vi "002 Case calculadora strings.vi"() -> ()   [LabVIEW 2019]
panel:
  out "Resultat":dbl
  in  "Selector d'operació":u8(slide) scale=0.0..3.0
  in  "Nombre 1":dbl
  in  "Nombre 2":dbl
  # "CALCULADORA"
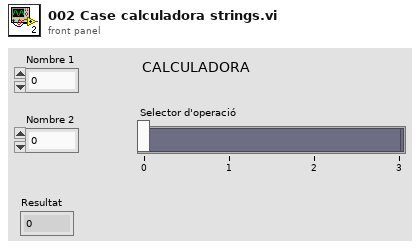
[diagram p1: front panel]
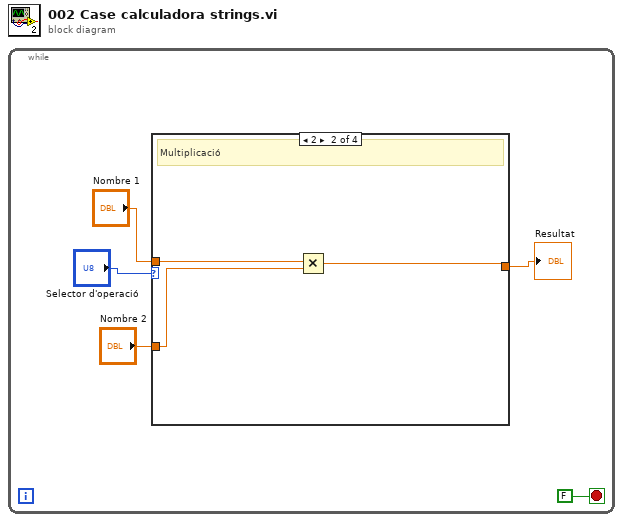
[diagram p0: block diagram]
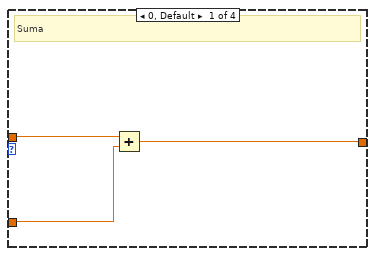
[diagram p2: hidden frame]
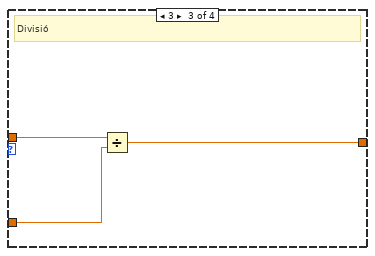
[diagram p3: hidden frame]
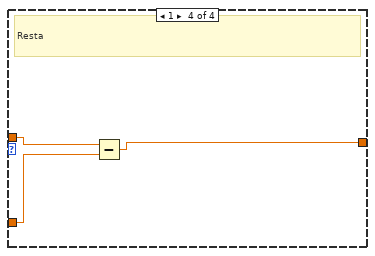
[diagram p4: hidden frame]
diagram:
  n1 = while {
    stop <- FALSE stop-if-true
    n2 = case shown="2" "Selector d'operació" {
      tunnel: "Nombre 1" -> [w8 w11 w14 w17]
      tunnel: "Nombre 2" -> [w7 w10 w13 w16]
      tunnel: [w6 w9 w12 w15] -> w2
      frame 0, Default {
        # "Suma"
        n3 = Add(x=w8, y=w7) -> (x+y=w6:dbl)
      }
      frame 2 {
        # "Multiplicació"
        n4 = Multiply(x=w11, y=w10) -> (x*y=w9:dbl)
      }
      frame 3 {
        # "Divisió"
        n5 = Divide(x=w14, y=w13) -> (x/y=w12:dbl)
      }
      frame 1 {
        # "Resta"
        n6 = Subtract(x=w17, y=w16) -> (x-y=w15:dbl)
      }
    }
    "Resultat" <- w2
  }
